vi "SetImpMode.vi"(8 "错误输入（无错误）":errorcluster, 10 "阻抗模式":u8) -> (0 "错误输出":errorcluster)   [LabVIEW 2018]
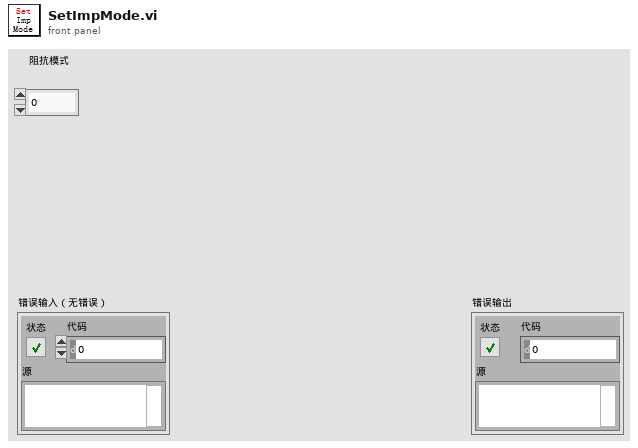
[diagram p1: front panel]
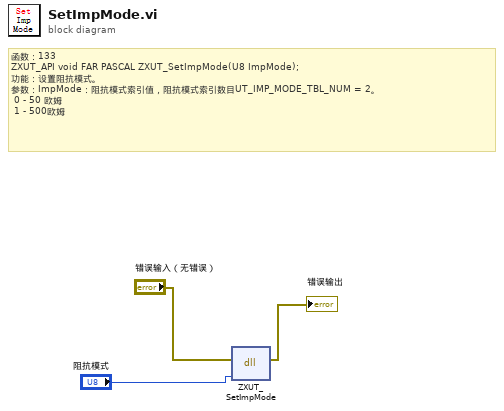
[diagram p0: block diagram]
diagram:
  # "函数：133\nZXUT_API void\tFAR PASCAL ZXUT_SetImpMode(U8 ImpMode);\n功能：设置阻抗模式。\n参数：ImpMode：阻抗模式索引值，阻抗模式索引数目UT_IMP_MODE_TBL_NUM = 2。\n\t0 - 50 欧姆\n\t1 - 500欧姆"
  n1 = dll-call lib="PTH2Rabs E软件项目超声超声子VI函数VI\tTCG处理ZXUTConfigMgr.dll" fn="ZXUT_SetImpMode"(error in="错误输入（无错误）", "ImpMode"="阻抗模式") -> (error out=→"错误输出":errorcluster)  [unwired: 4 in, 1 out]
